vi "open.vi"(8 "error in (no error)":errorcluster, 11 "Instrument in":refnum<class "Lock-In Amplifier.lvclass">) -> (0 "error out":errorcluster, 3 "Instrument out":refnum<class "Lock-In Amplifier.lvclass">)   [LabVIEW 2020, in "Lock-In Amplifier.lvclass"]
uses:
  Lock-In Amplifier.lvclass
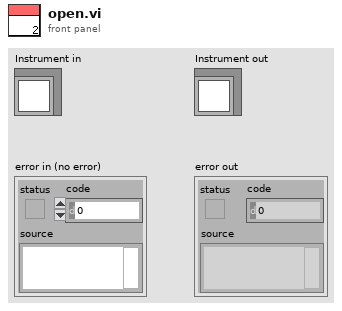
[diagram p1: front panel]
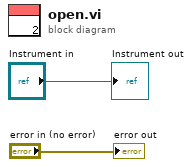
[diagram p0: block diagram]
diagram:
  "error out" <- "error in (no error)"
  "Instrument out" <- "Instrument in"
